vi "Route Signal by Name.vi"(8 "error in":errorcluster, 9 "Destination":string, 10 "Source":string, 11 "2525 in":refnum<class "2525.lvclass">) -> (0 "error out":errorcluster, 3 "2525 out":refnum<class "2525.lvclass">)   [LabVIEW 2019, in "2525.lvlib" / "2525.lvclass"]
uses:
  Library/2525.lvclass
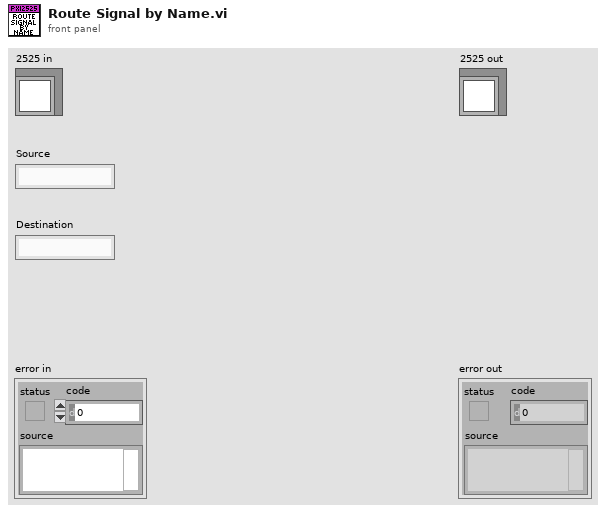
[diagram p1: front panel]
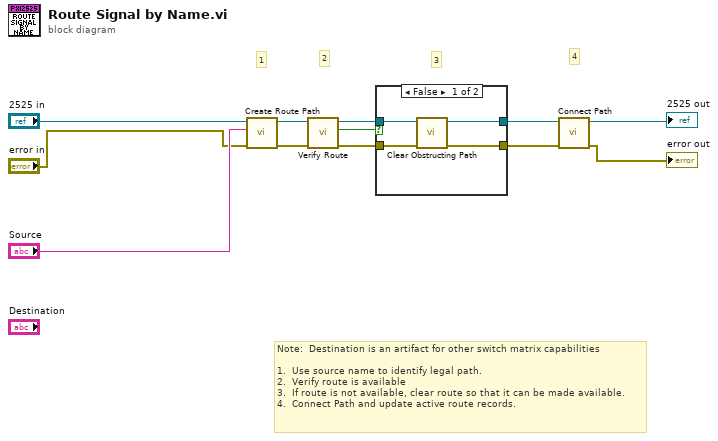
[diagram p0: block diagram]
diagram:
  # "4"
  # "3"
  # "2"
  # "1"
  # "Note:  Destination is an artifact for other switch matrix capabilities\n\n1.  Use source name to identify legal path.\n2.  Verify route is available\n3.  If route is not available, clear route so that it can be made available.\n4.  Connect Path and update active route records."
  n1 = call "Create Route Path.vi"("error in"="error in", "Source"="Source", "2525 in"="2525 in") -> ("error out"=w7:errorcluster, "2525 out"=w6:refnum<class "2525.lvclass">)  [unwired: 7 in]
  n2 = call "Verify Route.vi"("error in"=w7, "2525 in"=w6) -> ("error out"=w3:errorcluster, "Can route?"=w5:bool, "2525 out"=w4:refnum<class "2525.lvclass">)  [unwired: 7 in]
  n3 = case shown="False" w5 {
    tunnel: w4 -> [w15 w18]
    tunnel: w3 -> [w16 w17]
    tunnel: [w14 w18] -> w1
    tunnel: [w13 w17] -> w2
    frame False {
      n4 = call "Clear Obstructing Path.vi"("error in"=w16, "2525 in"=w15) -> ("error out"=w13:errorcluster, "2525 out"=w14:refnum<class "2525.lvclass">)  [unwired: 8 in]
    }
    frame True {
    }
  }
  n5 = call "Connect Path.vi"("error in"=w2, "2525 in"=w1) -> ("error out"=→"error out":errorcluster, "2525 out"=→"2525 out":refnum<class "2525.lvclass">)  [unwired: 8 in]
